vi "acquireFixation.vi"(7 "file cluster":T1, 8 "Timeout":dbl=1500.0, 9 "Fixation time":dbl=200.0, 10 "Params":dbl[](array[numeric])=[0.0, 1.0, 0.0, 1.0], 11 "Location":dbl[](array[numeric])=[0.0, 0.0, 10.0]) -> (0 "Distance from center":dbl, 2 "Raw voltage samples":dbl[][](array[numeric]), 3 "Success":bool, 5 "output cluster":T1)   [LabVIEW 2010, in "Core SubVIs.lvlib"]
doc: "This VI loops for the timeout time until the location of the eye (adjusted with parameters by convertEye) is within the fixation radius for fixation time. The location array is [x,y,radius]. The params is [xoffset, xgain, yoffset, ygain]."
uses:
  Core SubVIs.lvlib
  Controls/TYPE - Count Time Method.ctl
  Controls/TYPE - Analog Data Queue Method.ctl
  <vilib>/imath/engines/lvmath2/RunTimeEngine/ErrorHandling/NIMS_Finalize Error.vi
  <vilib>/imath/engines/lvmath2/RunTimeEngine/NodeEndStatement/NIMS_NodeEndStatement_Output.vi
  <instcachedir>/0/NIMS_NodeEndStatement_Output_53EC0D466D134D7ABD903AC30B43404B.lvgen/NIMS_NodeEndStatement_Output_53EC0D466D134D7ABD903AC30B43404B_001.vi
  <instcachedir>/0/NIMS_NodeEndStatement_Output_53EC0D466D134D7ABD903AC30B43404B.lvgen/NIMS_NodeEndStatement_Output_53EC0D466D134D7ABD903AC30B43404B_009.vi
  <vilib>/imath/engines/lvmath2/RunTimeEngine/ArithmeticOperatorToken/NIMS_ArithmeticOperator_plus.vi
  <instcachedir>/0/NIMS_ArithmeticOperator_plus_5FA379184E244F92A148919B9FCD7B31.lvgen/NIMS_ArithmeticOperator_plus_5FA379184E244F92A148919B9FCD7B31_004.vi
  <vilib>/imath/engines/lvmath2/RunTimeEngine/BuiltInFunctions/mean/NIMS_CS=mean(CV,I32).vi
  <vilib>/imathl/engines/lvmath/Functions/Error Handling/Create Error.vi
  HDF5/HDF5.lvlib
panel:
  out "Vertical":waveform(dbl)(graph)
  out "Horizontal":waveform(dbl)(graph)
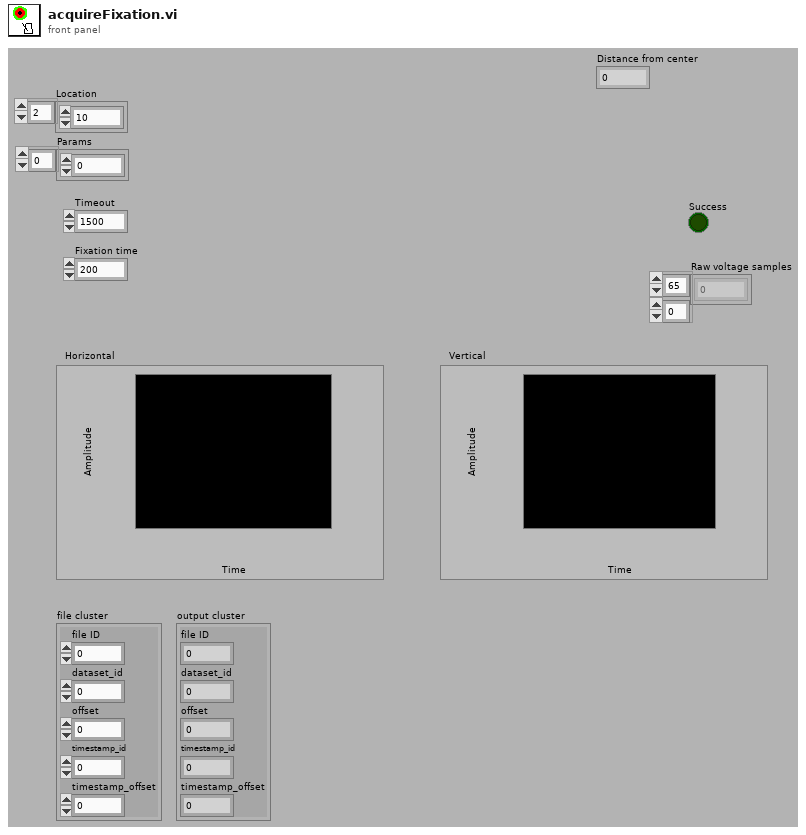
[diagram p1: front panel]
types:
  T1 = cluster{"file ID":i32, "dataset_id":i32, "offset":dbl, "timestamp_id":i32, "timestamp_offset":dbl}
  T2 = typedef "Core SubVIs.lvlib/TYPE - Count Time Method.ctl" = enum16{"Start Timer Task", "Read Timer", "Reset Timer", "Clear Timer Task"}
  T3 = typedef "Core SubVIs.lvlib/TYPE - Analog Data Queue Method.ctl" = enum16{"Set Data Queue", "Preview Element", "Remove Element", "Get Data Queue", "Flush Data Queue"}
  T4 = typedef "Core SubVIs.lvlib/TYPE - Analog Data.ctl" = waveform(dbl)[]
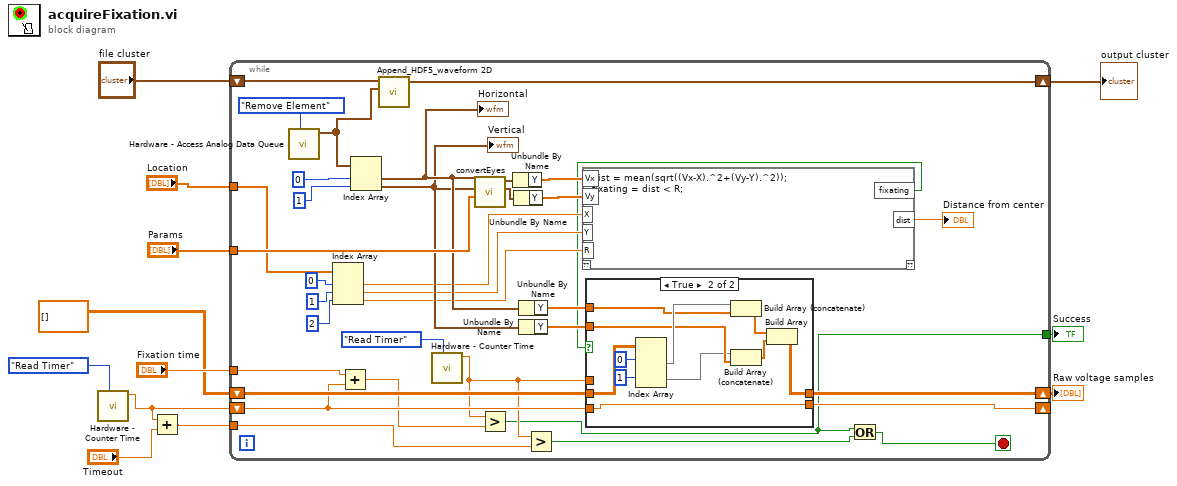
[diagram p0: block diagram]
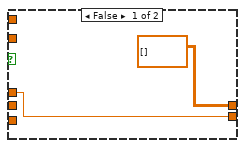
[diagram p2: hidden frame]
diagram:
  n1 = call "Hardware - Counter Time.vi"("Counter Time Function (Read Timer)"=TYPE_-_Count_Time_Method."Read Timer") -> ("Timer Value (ms)"=w7:dbl)  [unwired: 2 in, 8 out]
  n2 = Add(x=w7, y="Timeout") -> (x+y=w8:dbl)
  n3 = while {
    tunnel: "Params" -> [w46]
    tunnel: "Location" -> [w41]
    tunnel: "Fixation time" -> [w31]
    shift-right: [w38] -> w3
    shift-left: dbl[][] [] -> [w35]
    shift-right: [w34] -> _
    shift-left: w7 -> [w30]
    tunnel: w8 -> [w32]
    tunnel: [w26] -> w5
    shift-right: [w22] -> w2
    shift-left: "file cluster" -> [w21]
    stop <- w25 stop-if-true
    n4 = call "Hardware - Access Analog Data Queue.vi"("Method"=TYPE_-_Analog_Data_Queue_Method."Remove Element") -> ("Analog Data"=w20:T4)  [unwired: 3 in, 7 out]
    n5 = Index Array(array=w41, index #1=0 ("index"), index #2=1 ("index"), index #3=2 ("index")) -> (element #1=w17:dbl, element #2=w16:dbl, element #3=w15:dbl)
    n6 = Add(x=w31, y=w30) -> (x+y=w28:dbl)
    n7 = Index Array(array=w20, index #1=0 ("index"), index #2=1 ("index")) -> (element #1=w24:waveform(dbl), element #2=w23:waveform(dbl))
    "Vertical" <- w23
    "Horizontal" <- w24
    n8 = call "Append_HDF5_waveform 2D.vi"("file cluster"=w21, "data"=w20) -> ("output cluster"=w22:T1)  [unwired: 2 in, 4 out]
    n9 = call "Hardware - Counter Time.vi"("Counter Time Function (Read Timer)"=TYPE_-_Count_Time_Method."Read Timer") -> ("Timer Value (ms)"=w29:dbl)  [unwired: 2 in, 8 out]
    n10 = call "convertEyes.vi"("Params"=w46, "Vertical"=w23, "Horizontal"=w24) -> ("Vertical Calibrated"=w39:waveform(dbl), "Horizontal Calibrated"=w40:waveform(dbl))  [unwired: 7 out]
    n11 = Greater?(x=w29, y=w28) -> (0:w26:bool)
    n12 = Unbundle By Name(w40) -> ("Y"=w19:dbl[])
    n13 = Unbundle By Name(w39) -> ("Y"=w18:dbl[])
    n14 = Unbundle By Name(w24) -> ("Y"=w37:dbl[])
    n15 = Unbundle By Name(w23) -> ("Y"=w36:dbl[])
    n16 = Greater?(x=w29, y=w32) -> (0:w27:bool)
    n17 = mathscript code="dist = mean(sqrt((Vx-X).^2+(Vy-Y).^2));\nfixating = dist < R;"("Vx"=w19, "Vy"=w18, "X"=w17, "Y"=w16, "R"=w15) -> ("fixating"=w14:bool, "dist"=→"Distance from center":dbl)  [unwired: 2 out]
    n18 = case shown="True" w14 {
      tunnel: [dbl[][] [] w51] -> w38
      tunnel: w37 -> [_ w56]
      tunnel: w36 -> [_ w55]
      tunnel: w35 -> [_ w60]
      tunnel: w30 -> [_ w61]
      tunnel: [w49 w61] -> w34
      tunnel: w29 -> [w49 _]
      frame False {
      }
      frame True {
        n19 = Index Array(array=w60, index (row) #1=0 ("index (row)"), index (row) #2=1 ("index (row)")) -> (element #1=w57:dbl[], element #2=w54:dbl[])  [unwired: 2 in]
        n20 = Build Array (concatenate)(w57, w56) -> (w53:dbl[])
        n21 = Build Array (concatenate)(w54, w55) -> (w52:dbl[])
        n22 = Build Array(w53, w52) -> (w51:dbl[][])
      }
    }
    n23 = Or(x=w26, y=w27) -> (x .or. y?=w25:bool)
  }
  "Success" <- w5
  "Raw voltage samples" <- w3
  "output cluster" <- w2
